vi "sv_Convert THD+N Results.vi"(0 "Residue Magnitudes":cluster{"X":dbl[], "Y":dbl[]}[](array[cluster]) {"X" format="%.2f"; "Y" format="%.2f"}, 5 "Total Magnitudes":cluster{"X":dbl[], "Y":dbl[]}[](array[cluster]) {"X" format="%.2f"; "Y" format="%.2f"}, 12 "desired units":T2) -> (3 "units":T1(array[cluster]), 4 "THD+N":cluster{"frequency":dbl[], "amplitude":dbl[]}[](array[cluster]) {"amplitude" format="%.2f"; "frequency" format="%.2f"}, 6 "SINAD":cluster{"frequency":dbl[], "amplitude":dbl[]}[](array[cluster]) {"amplitude" format="%.2f"; "frequency" format="%.2f"})   [LabVIEW 2017, in "SoundVib_ContSweptSine.lvlib"]
uses:
  <vilib>/addons/Sound and Vibration/svt_Continuous Swept Sine/SoundVib_ContSweptSine.lvlib
  <vilib>/addons/Sound and Vibration/svt_Distortion/SoundVib_Distortion.lvlib
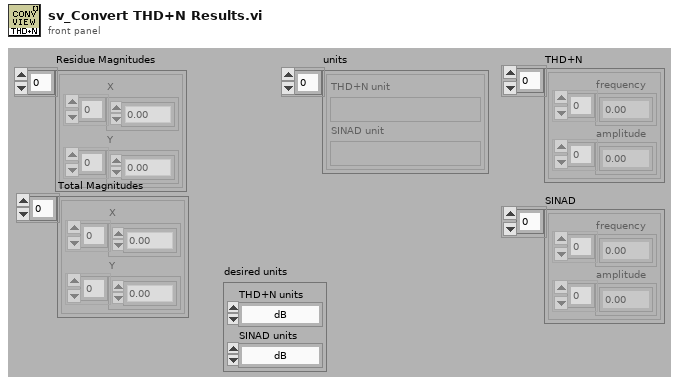
[diagram p1: front panel]
types:
  T1 = cluster{"THD+N unit":string, "SINAD unit":string}[]
  T2 = cluster{"THD+N units":enum16{"dB", "linear ratio", "%"}, "SINAD units":enum16{"dB", "linear ratio", "%"}}
  T3 = cluster{"unit label":string, "unit label":string}
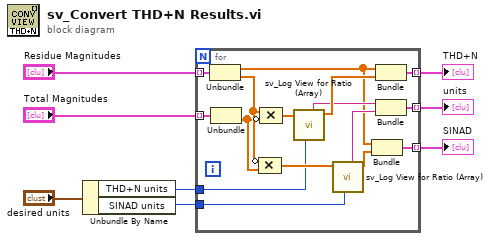
[diagram p0: block diagram]
diagram:
  n1 = Unbundle By Name("desired units") -> ("THD+N units"=w5:enum16{"dB", "linear ratio", "%"}, "SINAD units"=w4:enum16{"dB", "linear ratio", "%"})
  n2 = for {
    tunnel: "Residue Magnitudes" -> [w24] mode=indexing
    tunnel: "Total Magnitudes" -> [w23] mode=indexing
    tunnel: [w21] -> w3 mode=indexing
    tunnel: [w14] -> w2 mode=indexing
    tunnel: [w11] -> w1 mode=indexing
    tunnel: w5 -> [w10]
    tunnel: w4 -> [w9]
    n3 = Unbundle(w24) -> ("X"=w12:dbl[], "Y"=w19:dbl[])
    n4 = Unbundle(w23) -> ("Y"=w18:dbl[])  [unwired: 1 out]
    n5 = Compound Arithmetic op=MULTIPLY(invert w19, w18) -> (w17:dbl[])
    n6 = Compound Arithmetic op=MULTIPLY(w19, invert w18) -> (w22:dbl[])
    n7 = call <vilib>:"sv_Log View for Ratio (Array).vi"("ratio units"=w10, "linear ratio"=w22) -> ("converted ratio"=w20:dbl[], "unit label"=w16:string)  [unwired: 7 in, 1 out]
    n8 = call <vilib>:"sv_Log View for Ratio (Array).vi"("ratio units"=w9, "linear ratio"=w17) -> ("converted ratio"=w13:dbl[], "unit label"=w15:string)  [unwired: 7 in, 1 out]
    n9 = Bundle("X"=w12, "converted ratio"=w13) -> (w11:cluster{"X":dbl[], "converted ratio":dbl[]})  [unwired: 1 in]
    n10 = Bundle("X"=w12, "converted ratio"=w20) -> (w21:cluster{"X":dbl[], "converted ratio":dbl[]})  [unwired: 1 in]
    n11 = Bundle("unit label"=w16, "unit label"=w15) -> (w14:T3)  [unwired: 1 in]
  }
  "THD+N" <- w3
  "SINAD" <- w1
  "units" <- w2
